vi "start phase.vi"(4 "array":string[][](array[string]), 6 "Cluster":T1, 8 "error in (no error)":errorcluster, 9 "Start":bool, 10 "index (row)":u16, 11 "Programming Logic in":refnum<class "Programming Logic.lvclass">) -> (0 "error out":errorcluster, 1 "Speed":string, 3 "Programming Logic out":refnum<class "Programming Logic.lvclass">, 5 "Temp":string, 7 "Time":string)   [LabVIEW 2014, in "Files Library.lvlib" / "Programming Logic.lvclass"]
uses:
  Programming Logic.lvclass
  Programming Logic.lvclass/Programming Logic.ctl
  Files Library.lvlib
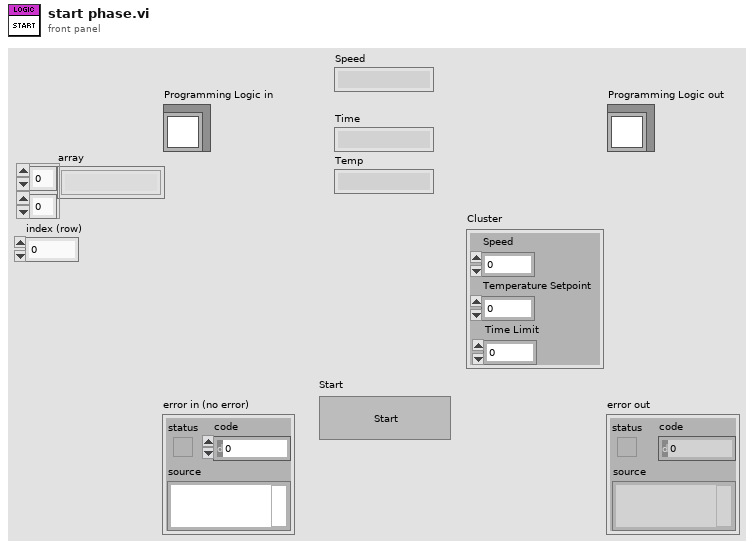
[diagram p1: front panel]
types:
  T1 = cluster{"Speed":u16, "Time Limit":u16, "Temperature Setpoint":u16}
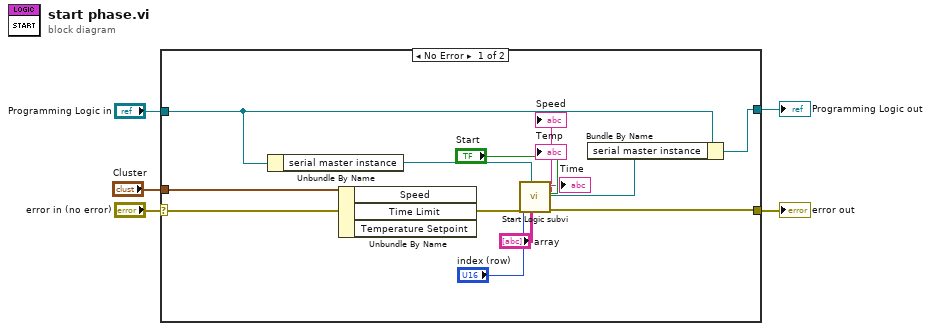
[diagram p0: block diagram]
diagram:
  n1 = case shown="No Error" "error in (no error)" {
    selector: "error in (no error)" -> [w17 w20]
    tunnel: [w16 w20] -> w4
    tunnel: [w13 w19] -> w2
    tunnel: "Programming Logic in" -> [w14 w19]
    tunnel: "Cluster" -> [w12 _]
    frame No Error {
      n2 = Unbundle By Name(w14) -> ("serial master instance"=w18:refnum<class "Modbus Master.lvclass">)
      n3 = Unbundle By Name(w12) -> ()  [unwired: 3 out]
      n4 = call "Start Logic subvi.vi"("Start"="Start", "Modbus master in"=w18, "array"="array", "error in"=w17, "index (row)"="index (row)") -> ("Modbus master out"=w15:refnum<class "Modbus Master.lvclass">, "error out"=w16:errorcluster, "Time"=→"Time":string, "Temp"=→"Temp":string, "Speed"=→"Speed":string)  [unwired: 2 in]
      n5 = Bundle By Name(cluster=w14, "serial master instance"=w15) -> (w13:refnum<class "Programming Logic.lvclass">)
    }
    frame Error {
    }
  }
  "error out" <- w4
  "Programming Logic out" <- w2
